vi "Get Screen Coordinates.vi"(8 "error in (no error)":errorcluster, 11 "Boolean in":refnum<vi>) -> (0 "error out":errorcluster, 3 "ScreenCoords":T1)   [LabVIEW 2012, in "Win8uiDemo.lvlib" / "Flyout.lvclass"]
uses:
  Flyout.lvclass
  <vilib>/Utility/miscctls.llb/LVPointTypeDef.ctl
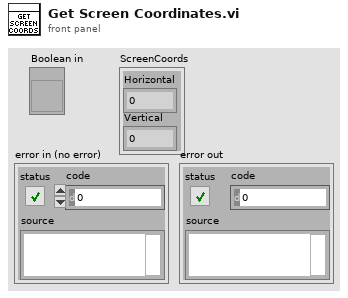
[diagram p1: front panel]
types:
  T1 = typedef "LVPointTypeDef.ctl" = cluster{"Horizontal":i16, "Vertical":i16}
  T2 = typedef "LVPositionTypeDef.ctl" = cluster{"Left":i32, "Top":i32}
  T3 = typedef "LVRectTypeDef.ctl" = cluster{"Left":i16, "Top":i16, "Right":i16, "Bottom":i16}
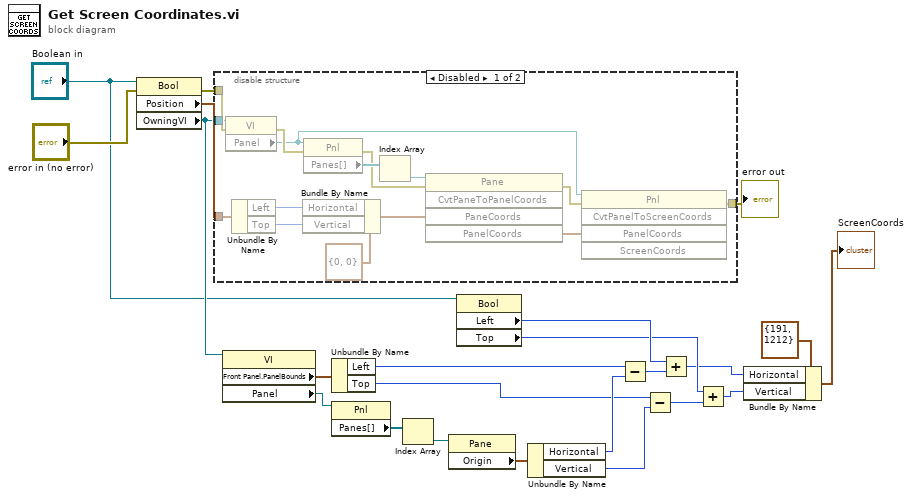
[diagram p0: block diagram]
diagram:
  n1 = property on="Property Node" class="Bool"(reference="Boolean in", error in="error in (no error)") -> (error out=w22:errorcluster, "Position"=w20:T2, "OwningVI"=w18:refnum<vi>)  [unwired: 1 out]
  n2 = disable-structure shown="Disabled" {
    disable-tunnel: w22 -> [w36 _]
    disable-tunnel: [w32 _] -> w21
    disable-tunnel: w20 -> [w31 _]
    disable-tunnel: w18 -> [w24 _]
    frame Disabled {
      n3 = property class="VI"(reference=w24, error in=w36) -> (error out=w35:errorcluster, "Panel"=w26:refnum<vi>)  [unwired: 1 out]
      n4 = Unbundle By Name(w31) -> ("Left"=w29:i32, "Top"=w28:i32)
      n5 = Bundle By Name(cluster=T1 {"Horizontal"=0, "Vertical"=0} ("Panel Coordinates"), "Horizontal"=w29, "Vertical"=w28) -> (w27:T1)
      n6 = property class="Pnl"(reference=w26, error in=w35) -> (error out=w34:errorcluster, "Panes[]"=w38:refnum<vi>[])  [unwired: 1 out]
      n7 = Index Array(array=w38) -> (element=w25:refnum<vi>)  [unwired: 1 in]
      n8 = invoke class="Pane" method="CvtPaneToPanelCoords"(reference=w25, error in=w34, "PaneCoords"=w27) -> (error out=w33:errorcluster, "PanelCoords"=w37:T1)  [unwired: 2 in, 3 out]
      n9 = invoke class="Pnl" method="CvtPanelToScreenCoords"(reference=w26, error in=w33, "PanelCoords"=w37) -> (error out=w32:errorcluster)  [unwired: 2 in, 4 out]
    }
    frame Enabled {
    }
  }
  "error out" <- w21
  n10 = property class="VI"(reference=w18) -> ("Front Panel.PanelBounds"=w17:T3, "Panel"=w15:refnum<vi>)  [unwired: 1 in, 2 out]
  n11 = Unbundle By Name(w17) -> ("Left"=w11:i16, "Top"=w9:i16)
  n12 = property class="Pnl"(reference=w15) -> ("Panes[]"=w16:refnum<vi>[])  [unwired: 1 in, 2 out]
  n13 = Index Array(array=w16) -> (element=w14:refnum<vi>)  [unwired: 1 in]
  n14 = property class="Pane"(reference=w14) -> ("Origin"=w13:T1)  [unwired: 1 in, 2 out]
  n15 = property class="Bool"(reference="Boolean in") -> ("Left"=w7:i32, "Top"=w4:i32)  [unwired: 1 in, 2 out]
  n16 = Unbundle By Name(w13) -> ("Horizontal"=w10:i16, "Vertical"=w8:i16)
  n17 = Subtract(x=w11, y=w10) -> (x-y=w6:i16)
  n18 = Subtract(x=w9, y=w8) -> (x-y=w5:i16)
  n19 = Add(x=w7, y=w6) -> (x+y=w3:i32)
  n20 = Add(x=w4, y=w5) -> (x+y=w2:i32)
  n21 = Bundle By Name(cluster=T1 {"Horizontal"=191, "Vertical"=1212} ("ScreenCoords"), "Horizontal"=w3, "Vertical"=w2) -> (→"ScreenCoords":T1)
